vi "Write Test Mode.vi"(8 "error in (no error)":errorcluster, 10 "Test Mode":string(combo), 11 "Post Analysis in":refnum<class "Post Analysis.lvclass">) -> (0 "error out":errorcluster, 3 "Post Analysis out":refnum<class "Post Analysis.lvclass">)   [LabVIEW 2023, in "Data Analysis.lvlib" / "Post Analysis.lvlib" / "Post Analysis.lvclass"]
uses:
  Post Analysis.lvclass
  Post Analysis.lvclass/Post Analysis.ctl
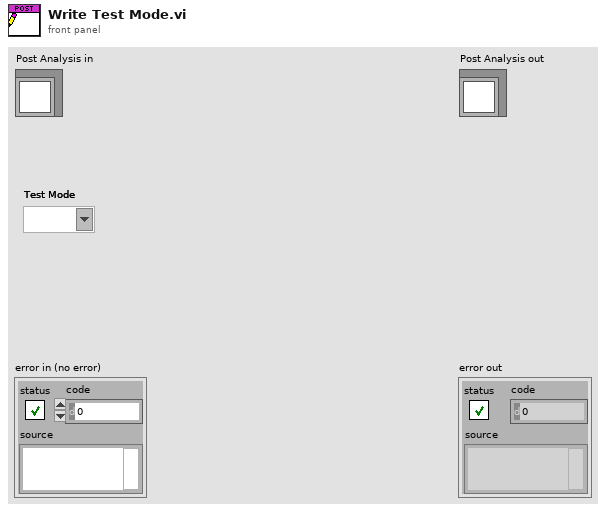
[diagram p1: front panel]
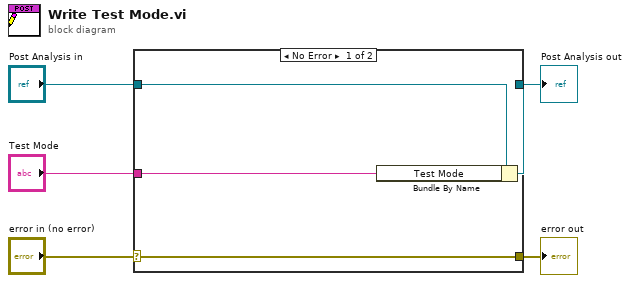
[diagram p0: block diagram]
diagram:
  n1 = case shown="No Error" "error in (no error)" {
    selector: "error in (no error)" -> [w9 w10]
    tunnel: [w9 w10] -> w4
    tunnel: [w7 w11] -> w2
    tunnel: "Post Analysis in" -> [w8 w11]
    tunnel: "Test Mode" -> [w6 _]
    frame No Error {
      n2 = Bundle By Name(cluster=w8, "Test Mode"=w6) -> (w7:refnum<class "Post Analysis.lvclass">)
    }
    frame Error {
    }
  }
  "error out" <- w4
  "Post Analysis out" <- w2
